vi "DCV_OneChannel.vi"(6 "LowLimit":dbl, 7 "HiLimit":dbl, 8 "Error In":errorcluster, 10 "Channel":string="101", 11 "VISA resource name":refnum<visa-resource-name>="COM5") -> (0 "Error Out":errorcluster, 1 "Value":string, 2 "number":dbl=1.33828, 3 "VISA resource name out":refnum<visa-resource-name>="COM5")   [LabVIEW 2013]
uses:
  <vilib>/Utility/error.llb/whitespace.ctl
panel:
  out "testlist":dbl[](array[numeric])=[1.33831, 1.33831, 1.33831, 1.33831, 1.3383, 1.3383, 1.3383, 1.3383, 1.33829, 1.33829, 1.33829, 1.33829, 1.33828, 1.33828, 1.33828, 1.33828]
  out "read buffer":string="SCAN OK\n"
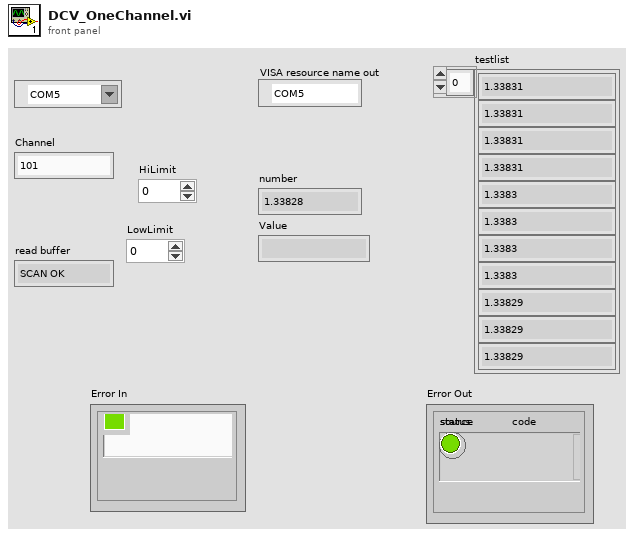
[diagram p1: front panel]
types:
  T1 = typedef "whitespace.ctl" = u16
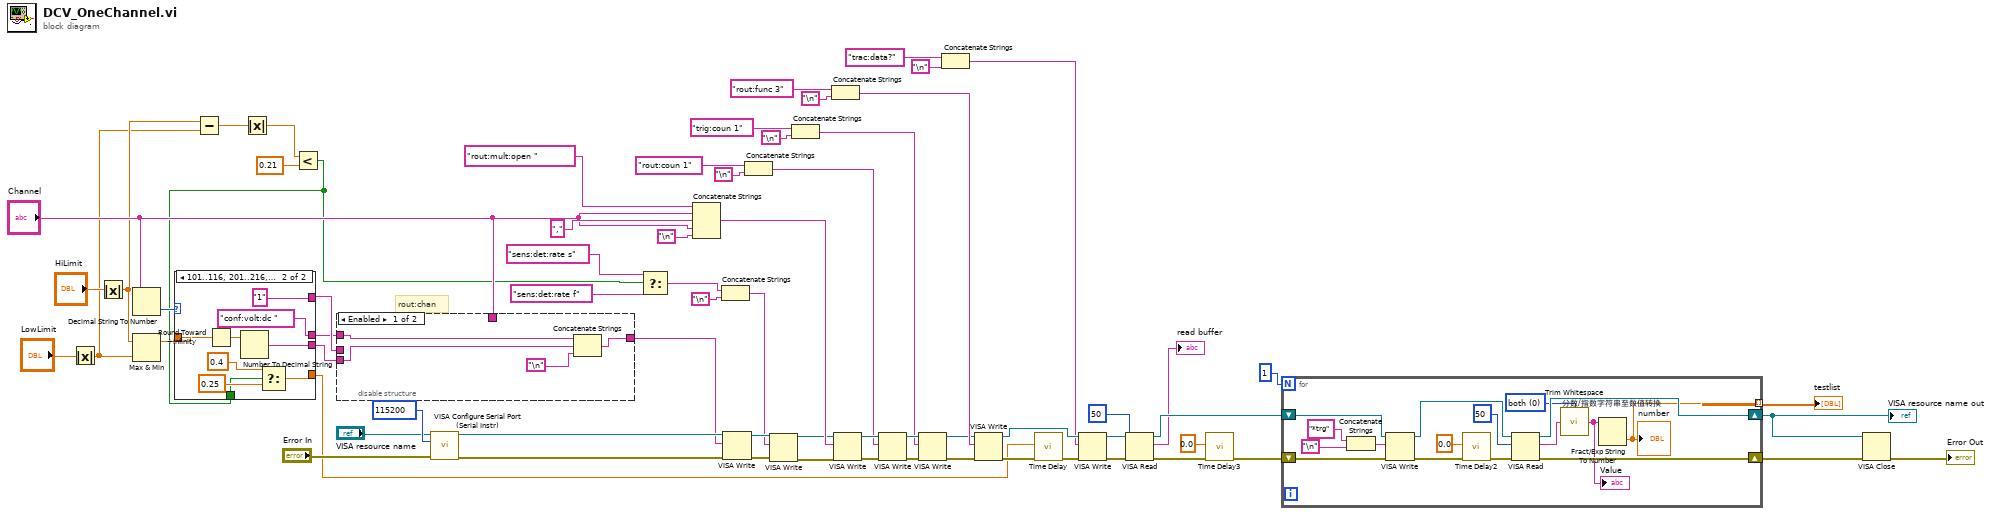
[diagram p0: block diagram]
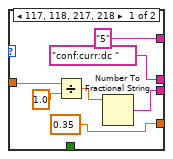
[diagram p2: hidden frame]
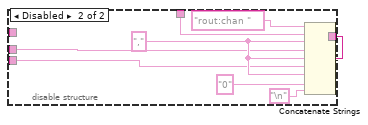
[diagram p3: hidden frame]
diagram:
  # "rout:chan"
  n1 = Absolute Value(x="LowLimit") -> (abs(x)=w8:dbl)
  n2 = Absolute Value(x="HiLimit") -> (abs(x)=w9:dbl)
  n3 = Decimal String To Number(string="Channel") -> (number=w22:i32)  [unwired: 2 in, 1 out]
  n4 = Max & Min(x=w9, y=w8) -> (max(x,y)=w19:dbl)  [unwired: 1 out]
  n5 = Subtract(x=w9, y=w8) -> (x-y=w7:dbl)
  n6 = Absolute Value(x=w7) -> (abs(x)=w6:dbl)
  n7 = Less?(x=w6, y=0.21) -> (x < y?=w1:bool)
  n8 = case shown="101..116, 201..216, Default" w22 {
    tunnel: ["5" "1"] -> w24
    tunnel: w19 -> [w73 w82]
    tunnel: [w70 w81] -> w18
    tunnel: ["conf:curr:dc " ("write buffer") "conf:volt:dc " ("write buffer")] -> w17
    tunnel: [0.35 ("wait scan") w76] -> w10
    tunnel: w1 -> [_ w77]
    frame 117, 118, 217, 218 {
      n9 = Divide(x=w73, y=1.0) -> (x/y=w71:dbl)
      n10 = Number To Fractional String(number=w71) -> (F-format string=w70:string)  [unwired: 3 in]
    }
    frame 101..116, 201..216, Default {
      n11 = Round Toward +Infinity(x=w82) -> (ceil(x): smallest int >= x=w83:dbl)
      n12 = Number To Decimal String(number=w83) -> (decimal integer string=w81:string)  [unwired: 1 in]
      n13 = Select(t=0.4 ("wait scan"), s=w77, f=0.25 ("wait scan")) -> (s? t:f=w76:dbl)
    }
  }
  n14 = disable-structure shown="Enabled" {
    disable-tunnel: [w88 w94] -> w64
    disable-tunnel: "Channel" -> [_ w95]
    disable-tunnel: w24 -> [_ w90]
    disable-tunnel: w18 -> [w87 w89]
    disable-tunnel: w17 -> [w85 _]
    frame Enabled {
      n15 = Concatenate Strings(w85, w87, "\n") -> (w88:string)
    }
    frame Disabled {
      w93 = ","
      n16 = Concatenate Strings("rout:chan " ("write buffer"), w95, w93, w90, w93, w89, w93, "0" ("string"), "\n") -> (w94:string)
    }
  }
  n17 = call <vilib>:"VISA Configure Serial Port (Serial Instr).vi"("VISA resource name"="VISA resource name", "baud rate (9600)"=u32 115200, "error in (no error)"="Error In") -> ("VISA resource name out"=w67:refnum<visa-resource-name>, "error out"=w68:errorcluster)  [unwired: 11 in]
  n18 = Select(t="sens:det:rate s" ("write buffer"), s=w1, f="sens:det:rate f" ("write buffer")) -> (s? t:f=w4:string)
  n19 = Concatenate Strings("rout:mult:open ", "Channel", ",", "Channel", "\n") -> (w61:string)
  n20 = Concatenate Strings(w4, "\n") -> (w11:string)
  n21 = VISA Write(VISA resource name=w67, write buffer=w64, error in (no error)=w68) -> (VISA resource name out=w15:refnum<visa-resource-name>, error out=w16:errorcluster)  [unwired: 1 out]
  n22 = Concatenate Strings("rout:coun 1" ("write buffer"), "\n") -> (w56:string)
  n23 = VISA Write(VISA resource name=w15, write buffer=w11, error in (no error)=w16) -> (VISA resource name out=w13:refnum<visa-resource-name>, error out=w14:errorcluster)  [unwired: 1 out]
  n24 = Concatenate Strings("trig:coun 1" ("write buffer"), "\n") -> (w51:string)
  n25 = Concatenate Strings("rout:func 3" ("write buffer"), "\n") -> (w48:string)
  n26 = VISA Write(VISA resource name=w13, write buffer=w61, error in (no error)=w14) -> (VISA resource name out=w59:refnum<visa-resource-name>, error out=w60:errorcluster)  [unwired: 1 out]
  n27 = VISA Write(VISA resource name=w59, write buffer=w56, error in (no error)=w60) -> (VISA resource name out=w54:refnum<visa-resource-name>, error out=w55:errorcluster)  [unwired: 1 out]
  n28 = VISA Write(VISA resource name=w54, write buffer=w51, error in (no error)=w55) -> (VISA resource name out=w26:refnum<visa-resource-name>, error out=w27:errorcluster)  [unwired: 1 out]
  n29 = Concatenate Strings("trac:data?" ("write buffer"), "\n") -> (w35:string)
  n30 = VISA Write(VISA resource name=w26, write buffer=w48, error in (no error)=w27) -> (VISA resource name out=w46:refnum<visa-resource-name>, error out=w47:errorcluster)  [unwired: 1 out]
  n31 = call "Time Delay"("error in (no error)"=w47, "Delay Time (s)"=w10) -> ("error out"=w34:errorcluster)  [unwired: 9 in]
  n32 = VISA Write(VISA resource name=w46, write buffer=w35, error in (no error)=w34) -> (VISA resource name out=w32:refnum<visa-resource-name>, error out=w33:errorcluster)  [unwired: 1 out]
  n33 = VISA Read(VISA resource name=w32, byte count=u32 50, error in (no error)=w33) -> (VISA resource name out=w44:refnum<visa-resource-name>, read buffer=→"read buffer":string, error out=w29:errorcluster)  [unwired: 1 out]
  n34 = call "Time Delay3"("error in (no error)"=w29, "Delay Time (s)"=0.0) -> ("error out"=w45:errorcluster)  [unwired: 9 in]
  n35 = for {
    N: 1 -> [_]
    shift-right: [w112] -> w66
    shift-left: w45 -> [w102]
    shift-right: [w111] -> w65
    shift-left: w44 -> [w101]
    tunnel: [w98] -> w25 mode=indexing
    w99 = T1 0 items=["both", "start of string", "end of string"] ("location (both)")
    n36 = Concatenate Strings("*trg" ("write buffer"), "\n") -> (w107:string)
    n37 = VISA Write(VISA resource name=w101, write buffer=w107, error in (no error)=w102) -> (VISA resource name out=w104:refnum<visa-resource-name>, error out=w106:errorcluster)  [unwired: 1 out]
    n38 = call "Time Delay2"("error in (no error)"=w106, "Delay Time (s)"=0.0) -> ("error out"=w105:errorcluster)  [unwired: 9 in]
    n39 = VISA Read(VISA resource name=w104, byte count=u32 50, error in (no error)=w105) -> (VISA resource name out=w111:refnum<visa-resource-name>, read buffer=w100:string, error out=w112:errorcluster)  [unwired: 1 out]
    n40 = call <vilib>:"Trim Whitespace.vi"("string"=w100, "location (both)"=w99) -> ("trimmed string"=w97:string)
    "Value" <- w97
    n41 = Fract/Exp String To Number "分数/指数字符串至数值转换"(string=w97) -> (number=w98:dbl)  [unwired: 3 in, 1 out]
    "number" <- w98
  }
  "VISA resource name out" <- w65
  "testlist" <- w25
  n42 = VISA Close(VISA resource name=w65, error in (no error)=w66) -> (error out=→"Error Out":errorcluster)
